vi "LWXPS_EventExtendedConfigurationActionSet.vi"(0 "Extended Action Name IN":string[](array[string]), 1 "Action Parameter 1 IN":string[](array[string]), 2 "Action Parameter 2 IN":string[](array[string]), 3 "Action Parameter 3 IN":string[](array[string]), 4 "Action Parameter 4 IN":string[](array[string]), 5 "LabVIEW error IN":errorcluster, 6 "XPS Reference IN":refnum<k24>) -> (10 "XPS Reference OUT":refnum<k24>, 12 "Returned error code":i32, 13 "LabVIEW error OUT":errorcluster, 14 "Extended Action Name OUT":string[](array[string]), 15 "Action Parameter 1 OUT":string[](array[string]), 16 "Action Parameter 2 OUT":string[](array[string]), 17 "Action Parameter 3 OUT":string[](array[string]), 18 "Action Parameter 4 OUT":string[](array[string]), 19 "XPS Error String":string)   [LabVIEW 2014]
uses:
  D:/XPSQ8_LabView_Library/Development/Source/Dll/Newport.XPS.CommandInterface.dll
  Dll/Newport.XPS.CommandInterface.dll
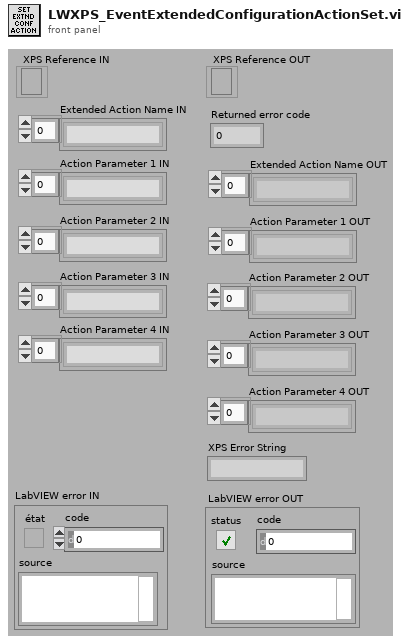
[diagram p1: front panel]
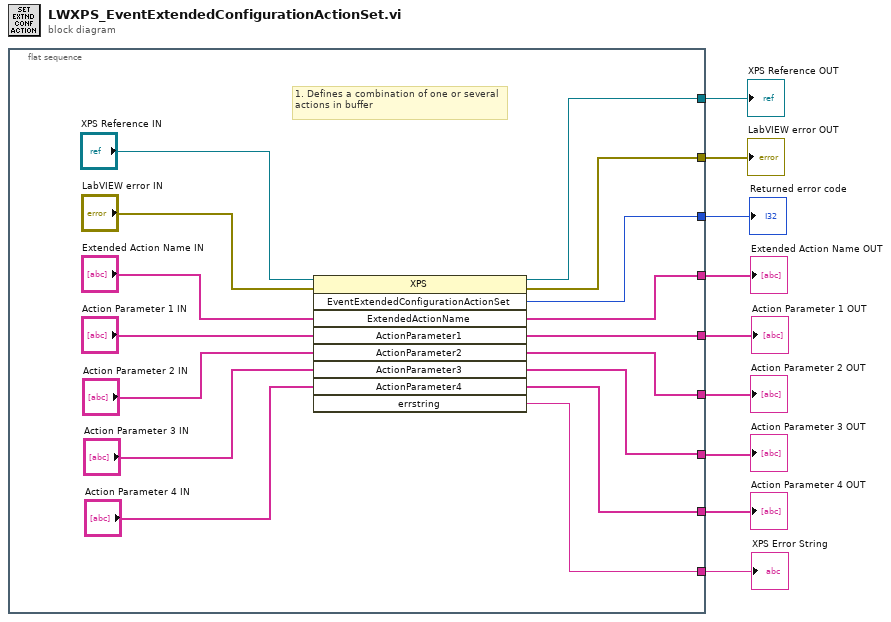
[diagram p0: block diagram]
diagram:
  n1 = flat-sequence {
    tunnel: [w20] -> w6
    tunnel: [w23] -> w9
    tunnel: [w22] -> w8
    tunnel: [w21] -> w7
    tunnel: [w13] -> w5
    tunnel: [w10] -> w4
    tunnel: [w17] -> w3
    tunnel: [w12] -> w2
    tunnel: [w11] -> w1
    frame #0 {
      # "1. Defines a combination of one or several actions in buffer"
      n2 = invoke class="XPS" method="EventExtendedConfigurationActionSet"(reference="XPS Reference IN", error in="LabVIEW error IN", "ExtendedActionName"="Extended Action Name IN", "ActionParameter1"="Action Parameter 1 IN", "ActionParameter2"="Action Parameter 2 IN", "ActionParameter3"="Action Parameter 3 IN", "ActionParameter4"="Action Parameter 4 IN") -> (reference out=w23:refnum<k24>, error out=w22:errorcluster, "EventExtendedConfigurationActionSet"=w21:i32, "ExtendedActionName"=w20:string[], "ActionParameter1"=w17:string[], "ActionParameter2"=w13:string[], "ActionParameter3"=w12:string[], "ActionParameter4"=w11:string[], "errstring"=w10:string)  [unwired: 2 in]
    }
  }
  "XPS Reference OUT" <- w9
  "LabVIEW error OUT" <- w8
  "Returned error code" <- w7
  "Extended Action Name OUT" <- w6
  "Action Parameter 2 OUT" <- w5
  "Action Parameter 3 OUT" <- w2
  "Action Parameter 4 OUT" <- w1
  "XPS Error String" <- w4
  "Action Parameter 1 OUT" <- w3
